vi "SupportedMetrics.vi"() -> (3 "Supported Metrics":string[](array[string]))   [LabVIEW 2017, in "AnalysisHelper.lvlib"]
uses:
  <vilib>/addons/InsightCM/Utilities/Analysis/Shared/AnalysisHelper.lvlib
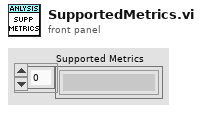
[diagram p1: front panel]
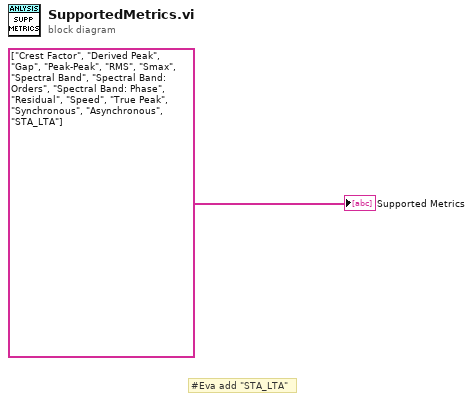
[diagram p0: block diagram]
diagram:
  # "#Eva add \"STA_LTA\""
  "Supported Metrics" <- string[] ["Crest Factor", "Derived Peak", "Gap", "Peak-Peak", "RMS", "Smax", "Spectral Band", "Spectral Band: Orders", "Spectral Band: Phase", "Residual", "Speed", "True Peak", "Synchronous", "Asynchronous", "STA_LTA"] ("value")
